vi "Demo_Andan get shift.vi"(10 "Time Stamp Out":timestamp[](array[timestamp])) -> (2 "Shift":i32)   [LabVIEW 2017]
panel:
  in  "Shift Time Details":T1 {"3End" format="%<%H:%M:%S\n%x>T"; "2End" format="%<%H:%M:%S\n%x>T"; "3Start" format="%<%H:%M:%S\n%x>T"; "2Start" format="%<%H:%M:%S\n%x>T"; "1End" format="%<%H:%M:%S\n%x>T"; "1Start" format="%<%H:%M:%S\n%x>T"}
  # "Start Time"
  # "End Time"
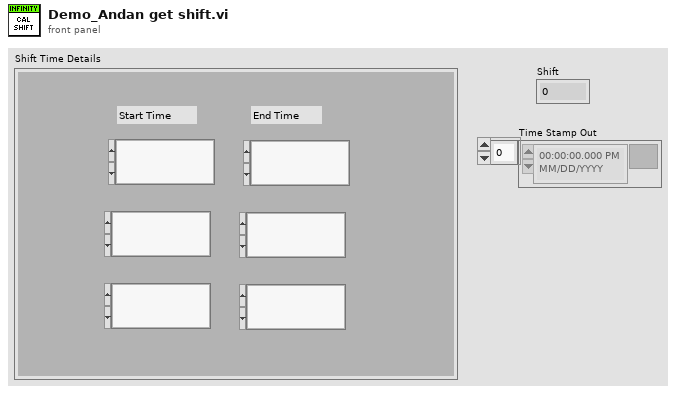
[diagram p1: front panel]
types:
  T1 = cluster{"1Start":timestamp, "1End":timestamp, "2Start":timestamp, "3Start":timestamp, "2End":timestamp, "3End":timestamp}
  T2 = typedef "LVDateTimeRec.ctl" = cluster{"fractional second":dbl, "second":i32, "minute":i32, "hour":i32, "day of month":i32, "month":i32, "year":i32, "day of week":i32, "day of year":i32, "DST":i32}
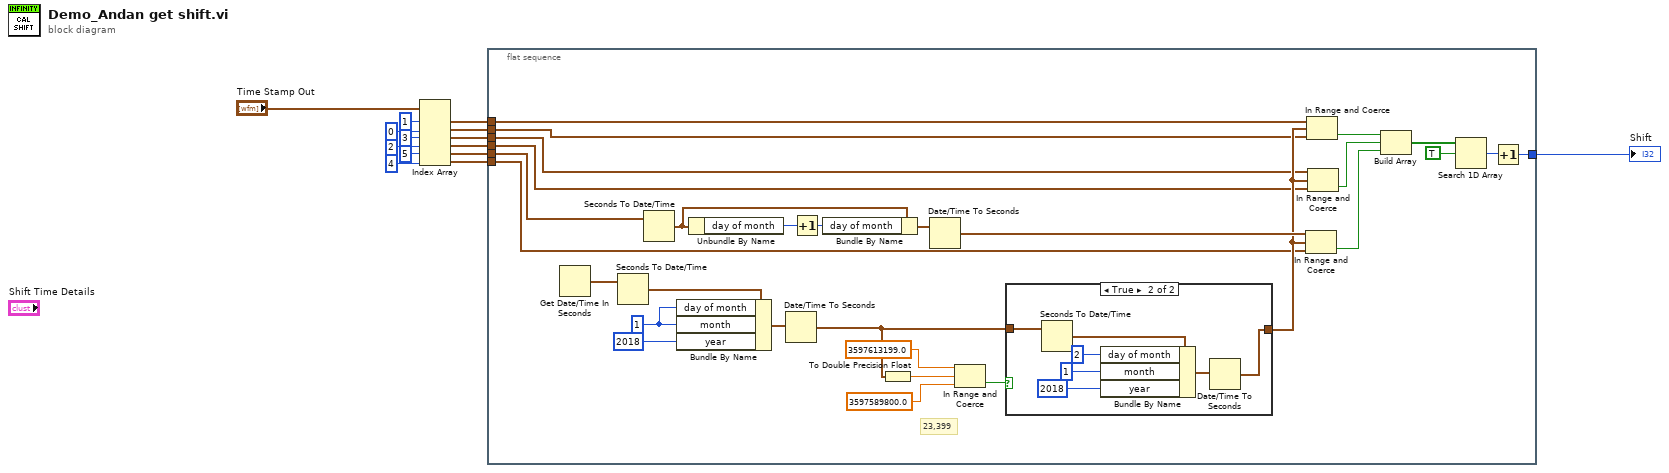
[diagram p0: block diagram]
diagram:
  n1 = Index Array(array="Time Stamp Out", index #1=1 ("index"), index #2=0 ("index"), index #3=3 ("index"), index #4=2 ("index"), index #5=5 ("index"), index #6=4 ("index")) -> (element #1=w10:timestamp, element #2=w9:timestamp, element #3=w6:timestamp, element #4=w5:timestamp, element #5=w2:timestamp, element #6=w1:timestamp)
  n2 = flat-sequence {
    tunnel: [w32] -> w14
    tunnel: w10 -> [w21]
    tunnel: w9 -> [w20]
    tunnel: w6 -> [w19]
    tunnel: w5 -> [w18]
    tunnel: w2 -> [w17]
    tunnel: w1 -> [w16]
    frame #0 {
      w25 = 1 ("day of month")
      # "23,399"
      n3 = Get Date/Time In Seconds() -> (seconds since 1Jan1904=w15:timestamp)
      n4 = Seconds To Date/Time(time stamp (now)=w15) -> (date time rec=w29:T2)  [unwired: 1 in]
      n5 = Seconds To Date/Time(time stamp (now)=w17) -> (date time rec=w42:T2)  [unwired: 1 in]
      n6 = Bundle By Name(cluster=w29, "day of month"=w25, "month"=w25, "year"=2018) -> (w31:T2)
      n7 = Unbundle By Name(w42) -> ("day of month"=w40:i32)
      n8 = Date/Time To Seconds(2:w31) -> (0:w23:timestamp)  [unwired: 1 in]
      n9 = Increment(x=w40) -> (x+1=w41:i32)
      n10 = Bundle By Name(cluster=w42, "day of month"=w41) -> (w43:T2)
      n11 = To Double Precision Float(number=w23) -> (double precision float=w26:dbl)
      n12 = Date/Time To Seconds(2:w43) -> (0:w39:timestamp)  [unwired: 1 in]
      n13 = In Range and Coerce(upper limit=3597613199.0 ("double precision float 2"), x=w26, lower limit=3597589800.0 ("double precision float")) -> (In Range?=w24:bool)  [unwired: 1 out]
      n14 = case shown="True" w24 {
        tunnel: w23 -> [w44 w47]
        tunnel: [w44 w46] -> w22
        frame False {
        }
        frame True {
          n15 = Seconds To Date/Time(time stamp (now)=w47) -> (date time rec=w49:T2)  [unwired: 1 in]
          n16 = Bundle By Name(cluster=w49, "day of month"=2, "month"=1 ("day of month"), "year"=2018) -> (w51:T2)
          n17 = Date/Time To Seconds(2:w51) -> (0:w46:timestamp)  [unwired: 1 in]
        }
      }
      n18 = In Range and Coerce(upper limit=w39, x=w22, lower limit=w16) -> (In Range?=w36:bool)  [unwired: 1 out]
      n19 = In Range and Coerce(upper limit=w21, x=w22, lower limit=w20) -> (In Range?=w38:bool)  [unwired: 1 out]
      n20 = In Range and Coerce(upper limit=w19, x=w22, lower limit=w18) -> (In Range?=w37:bool)  [unwired: 1 out]
      n21 = Build Array(w38, w37, w36) -> (w35:bool[])
      n22 = Search 1D Array(1D array=w35, element=TRUE) -> (index of element=w33:i32)  [unwired: 1 in]
      n23 = Increment(x=w33) -> (x+1=w32:i32)
    }
  }
  "Shift" <- w14
